vi "Test Worker Registered with Set Worker Handler.vi"(8 "error in (no error)":errorcluster, 11 "Worker Test in":refnum<class "Worker Test.lvclass">) -> (0 "error out":errorcluster, 3 "Worker Test out":refnum<class "Worker Test.lvclass">)   [LabVIEW 2020, in "Worker Test.lvclass"]
uses:
  Worker Test.lvclass
  C:/Program Files (x86)/National Instruments/LabVIEW 2020/vi.lib/Astemes/LUnit/Test Case.lvclass
  Test Doubles/Mock Job Handler/Mock Job Handler.lvclass
  C:/git/astemes-triarc-examples/source/Coffee Shop/Processes/People/Process Job/Job Handler.lvclass
  <vilib>/Astemes/Triarc Framework/Process/Process.lvclass/Process.ctl
  <vilib>/Astemes/LUnit/Test Case.lvclass/Test Case.ctl
  <vilib>/Astemes/Triarc Framework/Process/Private/SubVIs/Wait for finish.vi
  <vilib>/Astemes/Triarc Framework/Process/Private/SubVIs/Set Lifecycle State.vi
  <vilib>/Astemes/Triarc Framework/Process/Protected/Messaging/Send Message.vi
  <vilib>/Astemes/Triarc Framework/Process/Public/Lifecycle/Get Lifecycle State.vi
  <vilib>/Astemes/LUnit/Append Pass Result.vi
  <vilib>/Astemes/LUnit/Append Fail Result.vi
  <vilib>/Astemes/Triarc Framework/Process/Private/SubVIs/Handle Debug Data.vi
  <vilib>/Utility/error.llb/Clear Errors.vi
  <vilib>/Astemes/Triarc Framework/Logging/Log Debug.vi
  <vilib>/AdvancedString/1D String Array to Delimited String.vi
  <vilib>/Utility/High Resolution Relative Seconds.vi
  Processes/People/Workers/Worker/Worker.lvclass
  C:/Program Files (x86)/National Instruments/LabVIEW 2020/vi.lib/Astemes/Triarc Framework/Process/Process.lvclass
  <vilib>/Utility/error.llb/Error Cluster From Error Code.vi
  <vilib>/Astemes/Triarc Framework/Process/Public/Read Name.vi
  <vilib>/Astemes/Triarc Framework/Callback/Callback.lvclass
  <vilib>/Astemes/Triarc Framework/Process/Process.lvclass
  <vilib>/Astemes/LUnit/Test Case.lvclass
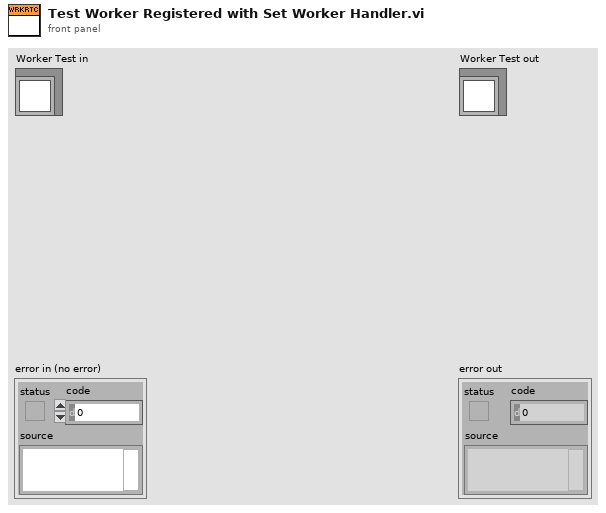
[diagram p1: front panel]
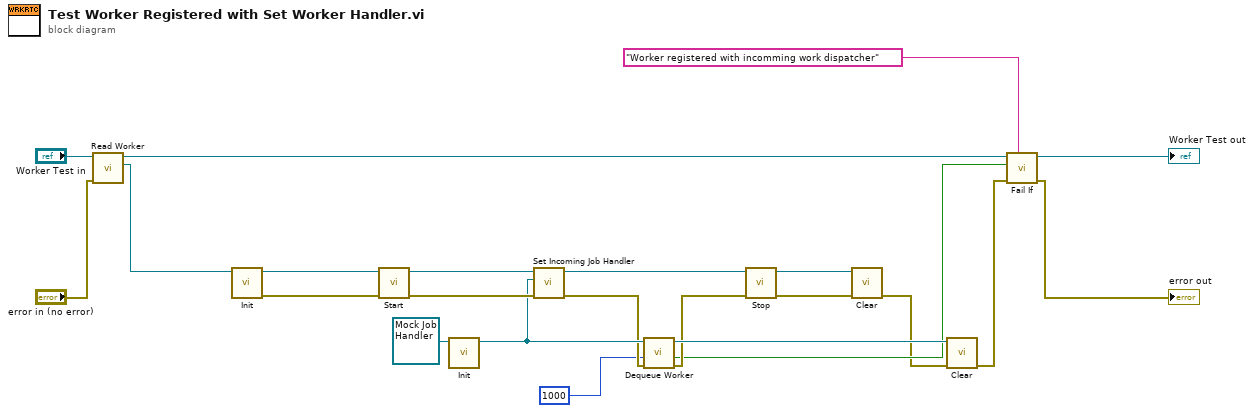
[diagram p0: block diagram]
diagram:
  n1 = call "Read Worker.vi"("error in (no error)"="error in (no error)", "Worker Test in"="Worker Test in") -> ("Worker"=w18:refnum<class "Worker.lvclass">, "Worker Test out"=w20:refnum<class "Worker Test.lvclass">)  [unwired: 7 in, 1 out]
  n2 = call-dynamic "Init.vi"("View In"=w18) -> ("error out"=w17:errorcluster, "View Out"=w14:refnum<class "Worker.lvclass">)  [unwired: 9 in]
  n3 = call <vilib>:"Start.vi"("error in (no error)"=w17, "Process In"=w14) -> ("error out"=w13:errorcluster, "Process Out"=w11:refnum<class "Worker.lvclass">)  [unwired: 7 in, 1 out]
  n4 = call-dynamic "Init.vi"("Mock Job Handler In"=refnum<class "Mock Job Handler.lvclass"> refnum ("Mock Worker In")) -> ("Mock Job Handler Out"=w8:refnum<class "Mock Job Handler.lvclass">)  [unwired: 9 in, 1 out]
  n5 = call "Set Incoming Job Handler.vi"("error in (no error)"=w13, "Job Handler"=w8, "Worker In"=w11) -> ("error out"=w6:errorcluster, "Worker Out"=w10:refnum<class "Worker.lvclass">)  [unwired: 7 in]
  n6 = call "Dequeue Worker.vi"("error in (no error)"=w6, "timeout in ms (-1)"=1000, "Mock Job Handler In"=w8) -> ("error out"=w5:errorcluster, "timed out?"=w3:bool, "Mock Job Handler Out"=w7:refnum<class "Mock Job Handler.lvclass">)  [unwired: 5 in, 1 out]
  n7 = call <vilib>:"Stop.vi"("error in (no error)"=w5, "Process In"=w10) -> ("error out"=w15:errorcluster, "Process Out"=w16:refnum<class "Worker.lvclass">)  [unwired: 7 in, 1 out]
  n8 = call-dynamic "Clear.vi"("error in (no error)"=w15, "View In"=w16) -> ("error out"=w2:errorcluster)  [unwired: 9 in]
  n9 = call-dynamic "Clear.vi"("error in (no error)"=w2, "Mock Job Handler In"=w7) -> ("error out"=w1:errorcluster)  [unwired: 9 in]
  n10 = call <vilib>:"Fail If.vi"("Description"="Worker registered with incomming work dispatcher", "error in (no error)"=w1, "Fail?"=w3, "LUnit Test Case In"=w20) -> ("error out"=→"error out":errorcluster, "LUnit Test Case Out"=→"Worker Test out":refnum<class "Worker Test.lvclass">)  [unwired: 6 in]
